vi "PositionTracer_Objects.vi"() -> ()   [LabVIEW 2012]
uses:
  <vilib>/vision/NI_Vision_Development_Module.lvlib
panel:
  in  "Settings":T1={"Objects"=0, "Threshold"=128, "Reject Border"=FALSE, "Fill Holes"=FALSE, "Min Object Size"=FALSE, "Min Size"=3, "Max Object Size"=FALSE, "Max Size"=100, "Show Search Area"=FALSE, "Show Center"=TRUE, "Show Bounding Box"=TRUE} {"Objects" items=["Bright Objects", "Dark Objects"]; "Threshold" min=1 max=999999999 step=1; "Max Size" min=1 max=999999999 step=1; "Min Size" min=1 max=999999999 step=1}
  in  "Pixel size Y":dbl=1.600000023841858
  in  "delay (s)":dbl=-0.9
  out "Y out chart":dbl(graph)
  out "X out chart":dbl(graph)
  out "Any missing frame?":bool
  out "Image":T2(plugin-control)
  in  "Tracking file":path=path "C:/Users/Ludovico/Lavoro/Experiments/Autofocus/vermi/track3.txt"
  in  "Pixel size X":dbl=1.600000023841858
  in  "Interframe time (s)":dbl=0.1
  in  "Image file pattern":string="*tif*"
  in  "Positions file":path=path "C:/Users/Ludovico/Lavoro/Experiments/Autofocus/vermi/CONFSTAGELOG/2016_12_16_10_06.txt"
  in  "Input images folder":path=path "C:/Users/Ludovico/Lavoro/Experiments/Autofocus/vermi/161216_1c_reduced"
  out "error out":errorcluster
  in  "error in (no error)":errorcluster
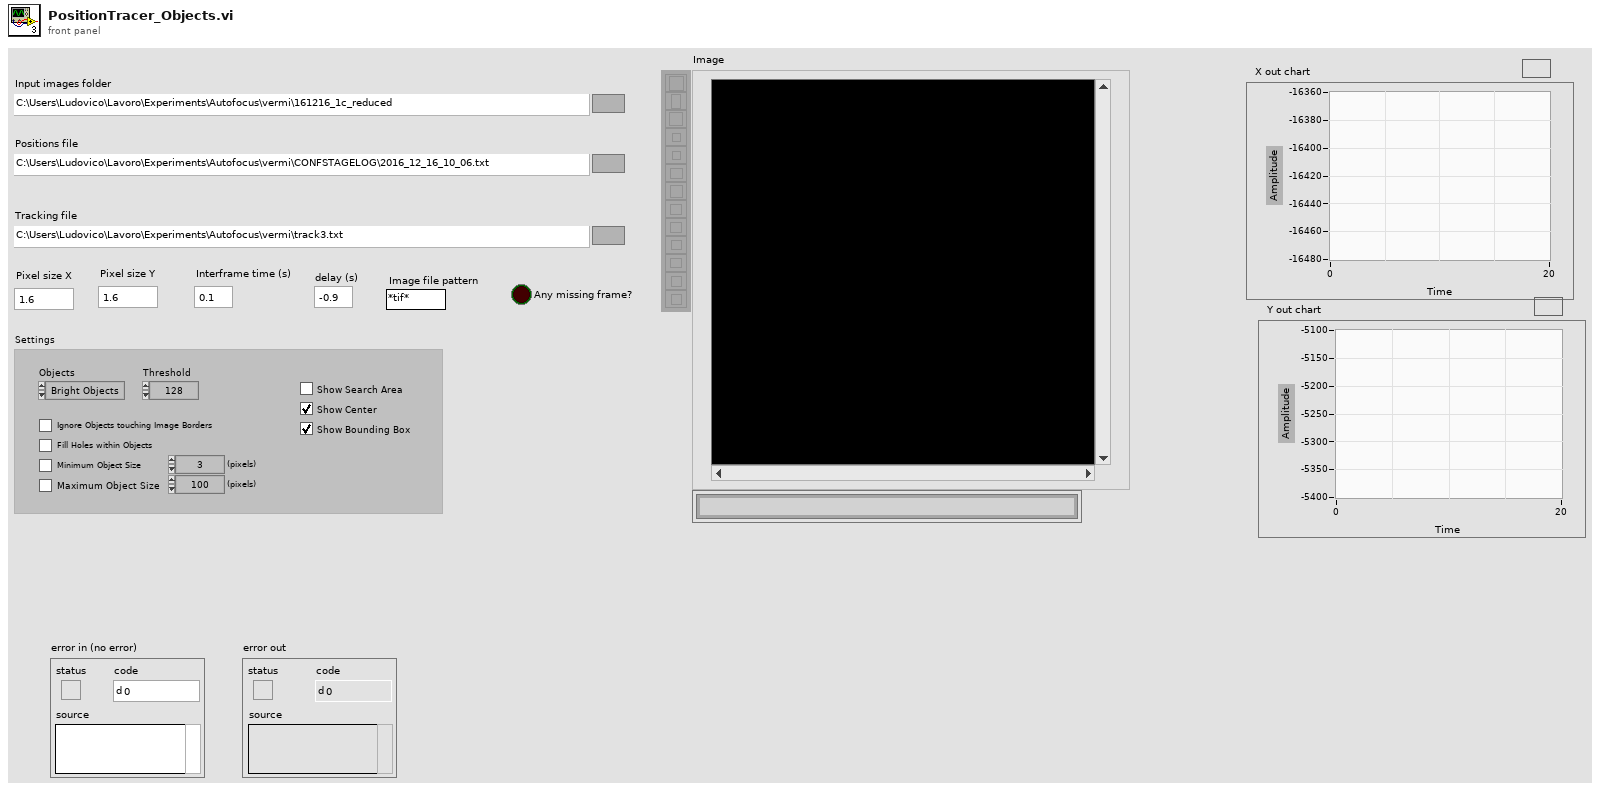
[diagram p1: front panel]
types:
  T1 = cluster{"Objects":u16, "Threshold":i32, "Reject Border":bool, "Fill Holes":bool, "Min Object Size":bool, "Min Size":i32, "Max Object Size":bool, "Max Size":i32, "Show Search Area":bool, "Show Center":bool, "Show Bounding Box":bool}
  T2 = typedef "IMAQ Image.ctl" = refnum<image>
  T3 = cluster{"X":dbl[], "Y":dbl[], "Focus":dbl[], "Time array":dbl[]}
  T4 = cluster{"Object Center":cluster{"X":sgl, "Y":sgl}, "Bounding Box":cluster{"X Left":i32, "Y Top":i32, "X Right":i32, "Y Bottom":i32}, "Area":sgl, "Orientation":sgl, "Aspect Ratio":sgl, "Nb Holes":i32}[]
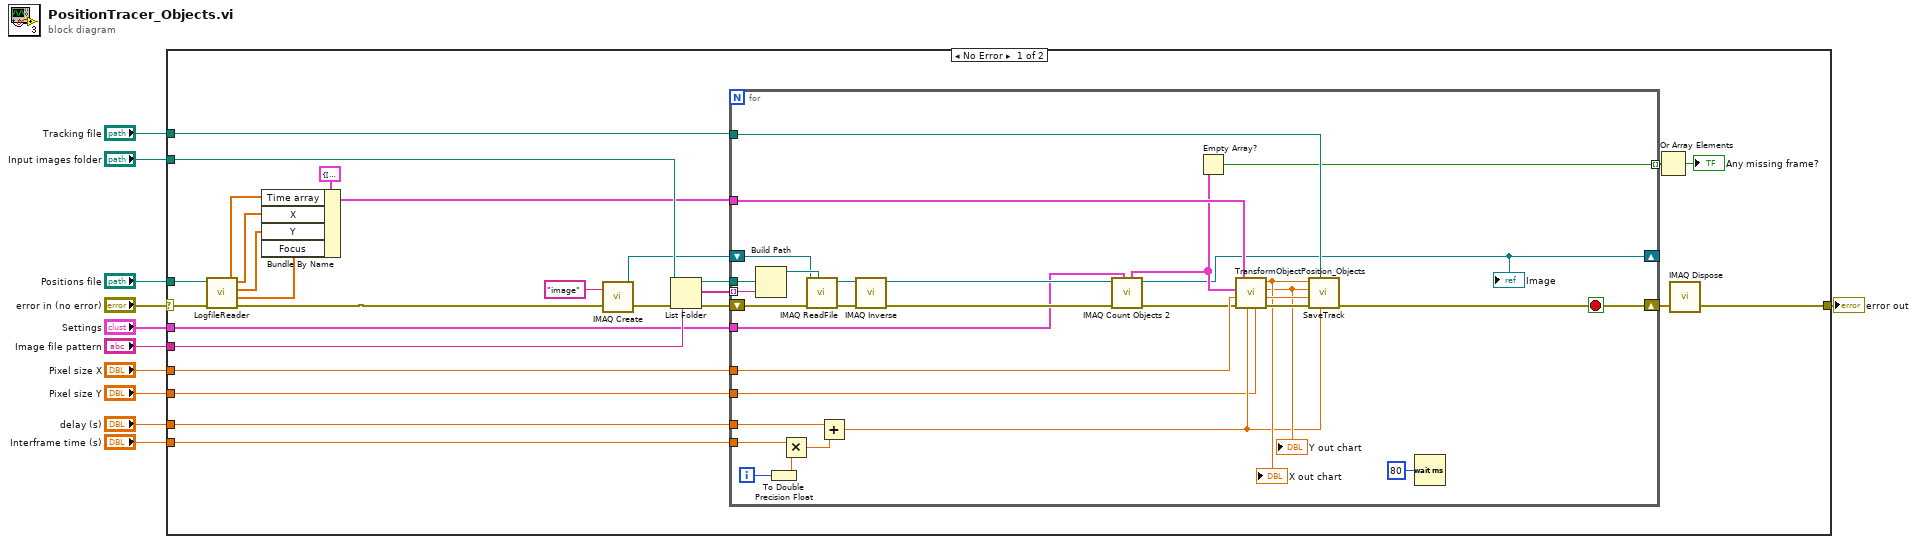
[diagram p0: block diagram]
diagram:
  n1 = case shown="No Error" "error in (no error)" {
    selector: "error in (no error)" -> [w38 w69]
    tunnel: "Positions file" -> [w35 _]
    tunnel: "Input images folder" -> [w34 _]
    tunnel: "Image file pattern" -> [w33 _]
    tunnel: "Interframe time (s)" -> [w22 _]
    tunnel: "Pixel size X" -> [w21 _]
    tunnel: "Tracking file" -> [w20 _]
    tunnel: [w13 w69] -> w4
    tunnel: "delay (s)" -> [w16 _]
    tunnel: "Pixel size Y" -> [w15 _]
    tunnel: "Settings" -> [w12 _]
    frame No Error {
      n2 = call "LogfileReader.vi"("error in (no error)"=w38, "Positions file"=w35) -> ("error out"=w14:errorcluster, "Focus"=w24:dbl[], "Y"=w25:dbl[], "X"=w26:dbl[], "Time"=w27:dbl[])  [unwired: 5 in]
      n3 = Bundle By Name(cluster=T3 {"X"=[], "Y"=[], "Focus"=[], "Time array"=[]} ("Spacetime cluster"), "Time array"=w27, "X"=w26, "Y"=w25, "Focus"=w24) -> (w23:T3)
      n4 = call "IMAQ Create"("Image Name"="image", "error in (no error)"=w14) -> ("New Image"=w29:T2, "error out"=w36:errorcluster)  [unwired: 3 in]
      n5 = List Folder(path=w34, pattern=w33, error in=w36) -> (path out=w30:path, filenames=w31:string[], error out=w32:errorcluster)  [unwired: 1 in, 1 out]
      n6 = for {
        tunnel: w31 -> [w67] mode=indexing
        tunnel: w30 -> [w66]
        shift-right: [w41] -> w19
        shift-left: w32 -> [w68]
        shift-right: [w40] -> _
        shift-left: w29 -> [w64]
        tunnel: w23 -> [w63]
        tunnel: w22 -> [w61]
        tunnel: w21 -> [w60]
        tunnel: w20 -> [w57]
        tunnel: [w55] -> w18 mode=indexing
        tunnel: w16 -> [w51]
        tunnel: w15 -> [w50]
        tunnel: w12 -> [w39]
        i -> [w48]
        stop <- w41 stop-if-true
        n7 = Build Path(base path=w66, name or relative path=w67) -> (appended path=w65:path)
        n8 = To Double Precision Float(number=w48) -> (double precision float=w62:dbl)
        n9 = Multiply(x=w61, y=w62) -> (x*y=w49:dbl)
        n10 = call "IMAQ ReadFile"("File Path"=w65, "error in (no error)"=w68, "Image"=w64) -> ("error out"=w47:errorcluster, "Image Out"=w46:T2)  [unwired: 4 in, 3 out]
        n11 = Add(x=w51, y=w49) -> (x+y=w52:dbl)
        n12 = call "IMAQ Inverse"("error in (no error)"=w47, "Image Src"=w46) -> ("error out"=w44:errorcluster, "Image Dst Out"=w43:T2)  [unwired: 8 in]
        n13 = call "IMAQ Count Objects 2"("Settings"=w39, "error in (no error)"=w44, "Image"=w43) -> ("error out"=w45:errorcluster, "Image Out"=w40:T2, "Objects"=w42:T4)  [unwired: 4 in, 2 out]
        "Image" <- w40
        n14 = Empty Array?(array=w42) -> (empty?=w55:bool)
        n15 = call "TransformObjectPosition_Objects.vi"("Pixel size Y"=w50, "Image time"=w52, "error in (no error)"=w45, "Pixel size X"=w60, "Objects"=w42, "Spacetime cluster"=w63) -> ("error out"=w59:errorcluster, "Focus out"=w58:dbl, "Y out"=w53:dbl, "X out"=w54:dbl)  [unwired: 2 in]
        "X out chart" <- w54
        "Y out chart" <- w53
        n16 = call "SaveTrack.vi"("Time"=w52, "Track file"=w57, "error in (no error)"=w59, "Focus"=w58, "Y"=w53, "X"=w54) -> ("error out"=w41:errorcluster)  [unwired: 5 in]
        n17 = Wait (ms)(milliseconds to wait=u32 80) -> ()  [unwired: 1 out]
      }
      n18 = Or Array Elements(Boolean array=w18) -> (logical OR=→"Any missing frame?":bool)
      n19 = call "IMAQ Dispose"("error in (no error)"=w19) -> ("error out"=w13:errorcluster)  [unwired: 5 in]
    }
    frame Error {
    }
  }
  "error out" <- w4
